vi "RecorderMainLoop.vi"(9 "NXT":T2={"Hardware"="NXT", "Flattened String"=""}, 13 "Terminate (Boolean CReference)":T1) -> (8 "NXT":T2={"Hardware"="NXT", "Flattened String"=""})   [LabVIEW 2010, in "Packet Recorder.lvlib"]
uses:
  Packet Recorder.lvlib
  <vilib>/NXT/Subs/LVHSConnector.ctl
  CLIB/CRef/Interface/CRef Boolean.llb/Boolean CReference.ctl
  CLIB/CRef/CRef.lvlib
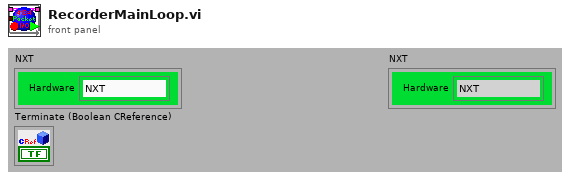
[diagram p1: front panel]
types:
  T1 = typedef "CRef.lvlib/Boolean CReference.ctl" = cluster{"Boolean CRef Address":u16, "Type":enum8{"Null", "Boolean", "U8", "I8", "U16", "I16", "U32", "I32", "U64", "I64", "Single", "Double", "Extended", "CSG", "CDB", "CXT", "Boolean(Def)"}}
  T2 = typedef "LVHSConnector.ctl" = cluster{"Hardware":string, "Flattened String":string}
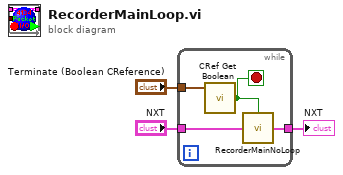
[diagram p0: block diagram]
diagram:
  n1 = while {
    tunnel: "NXT" -> [w6]
    tunnel: [w5] -> w2
    tunnel: "Terminate (Boolean CReference)" -> [w4]
    stop <- w7 stop-if-true
    n2 = call "CRef Get Boolean.vi"("Boolean CReference"=w4) -> ("Value"=w7:bool)  [unwired: 3 in, 1 out]
    n3 = call "RecorderMainNoLoop.vi"("NXT"=w6, "Close File? (False)"=w7) -> ("NXT"=w5:T2)
  }
  "NXT" <- w2
